vi "RichToFlatniswitch_grpc_GetRelayCountResponse.vi"(5 "OutputClusterType":T1, 11 "InputCluster":T2) -> (3 "OutputCluster":T1)   [LabVIEW 2021, in "NI Switch_client.lvlib"]
uses:
  NI Switch_client.lvlib
  niswitch_grpc_GetRelayCountResponse_Flat.ctl
  niswitch_grpc_GetRelayCountResponse.ctl
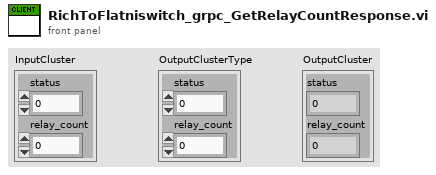
[diagram p1: front panel]
types:
  T1 = typedef "NI Switch_client.lvlib/niswitch_grpc_GetRelayCountResponse_Flat.ctl" = cluster{"status":i32, "relay_count":i32}
  T2 = typedef "NI Switch_client.lvlib/niswitch_grpc_GetRelayCountResponse.ctl" = cluster{"status":i32, "relay_count":i32}
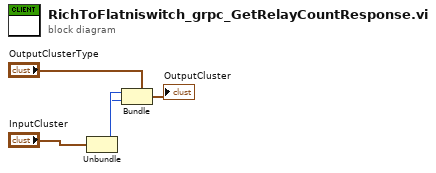
[diagram p0: block diagram]
diagram:
  n1 = Unbundle "Unbundle"("InputCluster") -> ("status"=w2:i32, "relay_count"=w1:i32)
  n2 = Bundle "Bundle"(cluster="OutputClusterType", "status"=w2, "relay_count"=w1) -> (→"OutputCluster":T1)
